vi "GFITS_Dhs_CmdHandling.vi"(0 "imname":string, 1 "fref":u64, 3 "filemsg":string, 5 "command":string, 7 "logfile":path, 9 "data":string, 11 "error in (no error)":errorcluster, 12 "expID":string, 13 "mext":bool, 14 "before expID":string) -> (2 "setref":bool, 4 "nodeID":string, 6 "response":string, 8 "fref out":u64, 10 "impath":string, 15 "error out":errorcluster)   [LabVIEW 2016]
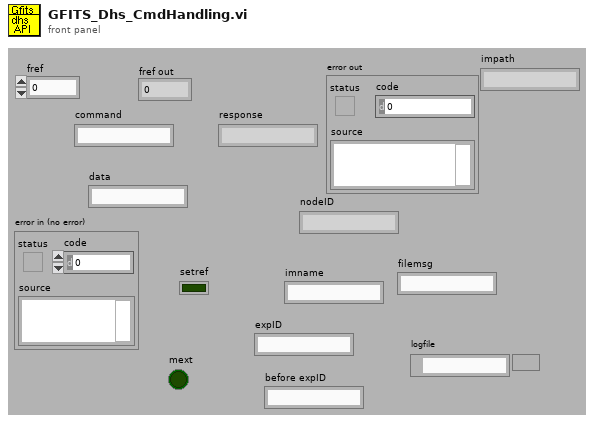
[diagram p1: front panel]
types:
  T1 = typedef "DatabaseHand_RefNum.ctl" = refnum<vi>
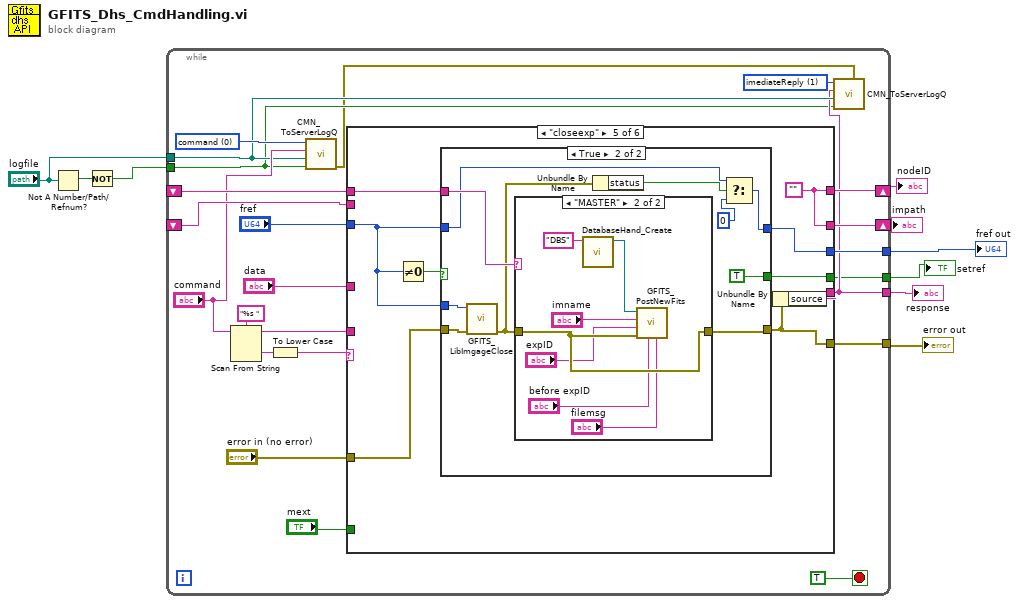
[diagram p0: block diagram]
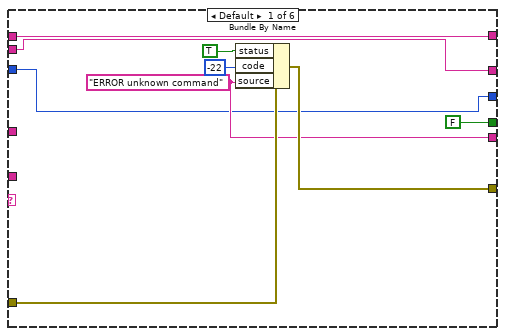
[diagram p2: hidden frame]
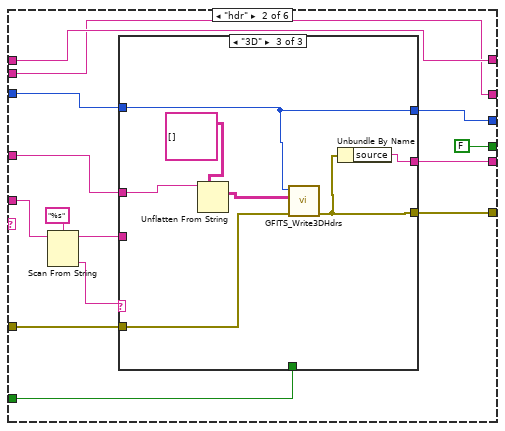
[diagram p3: hidden frame]
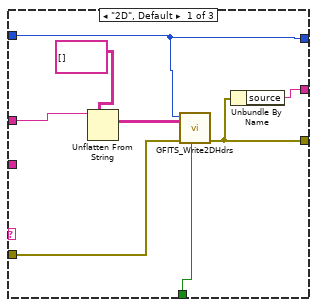
[diagram p4: hidden frame]
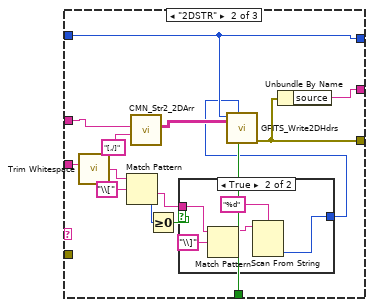
[diagram p5: hidden frame]
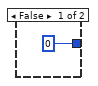
[diagram p6: hidden frame]
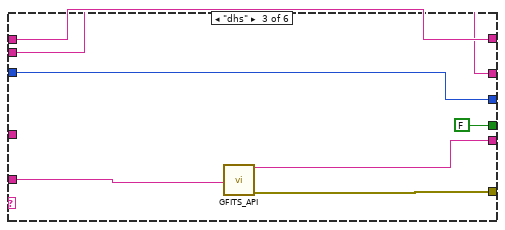
[diagram p7: hidden frame]
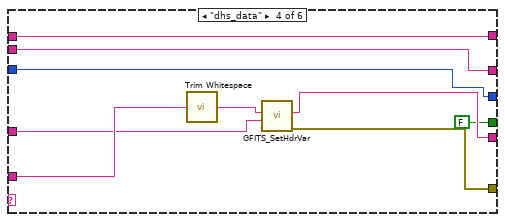
[diagram p8: hidden frame]
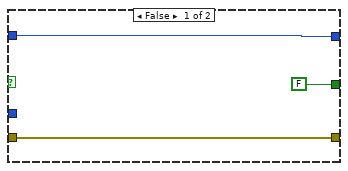
[diagram p9: hidden frame]
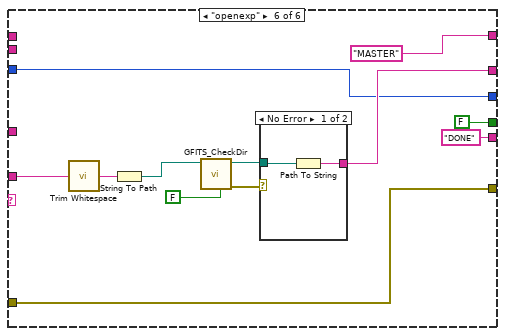
[diagram p11: hidden frame]
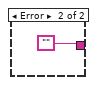
[diagram p12: hidden frame]
diagram:
  n1 = Not A Number/Path/Refnum?(number/path/refnum="logfile") -> (NaN/Path/Refnum?=w4:bool)
  n2 = Not(x=w4) -> (.not. x?=w2:bool)
  n3 = while {
    tunnel: [w26] -> w9
    tunnel: [w13] -> w8
    shift-right: [w23] -> w7
    shift-left: _ -> [w22]
    shift-right: [w21] -> w6
    shift-left: _ -> [w20]
    tunnel: [w19] -> w5
    tunnel: "logfile" -> [w15]
    tunnel: w2 -> [w12]
    tunnel: [w10] -> w1
    stop <- TRUE stop-if-true
    w14 = u16 1 items=["command", "imediateReply", "Callback Reply", "Information", "none"] ("type")
    w17 = u16 0 items=["command", "imediateReply", "Callback Reply", "Information", "none"] ("type")
    n4 = Scan From String(format string="%s ", input string="command") -> (remaining string=w29:string, output 1=w32:string)  [unwired: 2 in, 3 out]
    n5 = To Lower Case(string=w32) -> (all lower case string=w30:string)
    n6 = call "CMN_ToServerLogQ.vi"("Log"=w12, "file"=w15, "string"="command", "type"=w17) -> ("error out"=w11:errorcluster)  [unwired: 2 in, 4 out]
    n7 = case shown="\"closeexp\"" w30 {
      tunnel: w29 -> [_ w53 w96 w105 _ w145]
      tunnel: "data" -> [_ w52 _ w100 _ _]
      tunnel: [w40 w51 w97 w104 w114 w147] -> w26
      tunnel: "error in (no error)" -> [w41 w50 _ _ w115 w147]
      tunnel: [w37 w49 w95 w101 w113 "DONE" ("source")] -> w13
      tunnel: "fref" -> [w34 w48 w92 w99 w109 w138]
      tunnel: [w36 w47 w94 w103 w111 "MASTER"] -> w23
      tunnel: w22 -> [w36 w47 w94 w103 w110 _]
      tunnel: [w35 w46 w93 w102 w111 w139] -> w21
      tunnel: w20 -> [w35 w46 w93 w102 _ _]
      tunnel: [w34 w45 w92 w99 w108 w138] -> w19
      tunnel: "mext" -> [_ w44 _ _ _ _]
      tunnel: [FALSE ("setref") FALSE ("setref") FALSE ("setref") FALSE ("setref") w107 FALSE ("setref")] -> w10
      frame Default {
        w37 = "ERROR unknown command" ("source")
        n8 = Bundle By Name(cluster=w41, "status"=TRUE, "code"=-22, "source"=w37) -> (w40:errorcluster)
      }
      frame "hdr" {
        n9 = Scan From String(format string="%s", input string=w53) -> (remaining string=w43:string, output 1=w54:string)  [unwired: 2 in, 3 out]
        n10 = case shown="\"3D\"" w54 {
          tunnel: w52 -> [w63 w77 w90]
          tunnel: [w59 w74 w86] -> w51
          tunnel: w48 -> [w57 w72 w84]
          tunnel: w50 -> [w60 _ w87]
          tunnel: [w58 w73 w85] -> w49
          tunnel: [w57 w72 w84] -> w45
          tunnel: w44 -> [w56 w71 _]
          tunnel: w43 -> [_ w70 _]
          frame "2D", Default {
            n11 = Unflatten From String(type=string[][] [], binary string=w63) -> (value=w61:string[][])  [unwired: 1 in, 4 out]
            n12 = call "GFITS_Write2DHdrs.vi"("mext"=w56, "error in (no error)"=w60, "keys"=w61, "fref"=w57) -> ("error out"=w59:errorcluster)  [unwired: 1 in, 6 out]
            n13 = Unbundle By Name(w59) -> ("source"=w58:string)
          }
          frame "2DSTR" {
            n14 = call <vilib>:"Trim Whitespace.vi"("string"=w70) -> ("trimmed string"=w69:string)  [unwired: 1 in]
            n15 = Match Pattern(string=w69, regular expression="\\[") -> (after substring=w65:string, offset past match=w67:i32)  [unwired: 3 out]
            n16 = call "CMN_Str2_2DArr.vi"("col separator"="[,/]", "multi line string in"=w77) -> ("array out"=w75:string[][])  [unwired: 9 out]
            n17 = Greater Or Equal To 0?(x=w67) -> (x >= 0?=w66:bool)
            n18 = case shown="True" w66 {
              tunnel: w65 -> [_ w83]
              tunnel: [0 w79] -> w64
              frame False {
              }
              frame True {
                n19 = Match Pattern(string=w83, regular expression="\\]") -> (before substring=w81:string)  [unwired: 4 out]
                n20 = Scan From String(format string="%d", input string=w81) -> (output 1=w79:i32)  [unwired: 2 in, 4 out]
              }
            }
            n21 = call "GFITS_Write2DHdrs.vi"("mext"=w71, "extension"=w64, "keys"=w75, "fref"=w72) -> ("error out"=w74:errorcluster)  [unwired: 1 in, 6 out]
            n22 = Unbundle By Name(w74) -> ("source"=w73:string)
          }
          frame "3D" {
            n23 = Unflatten From String(type=string[][][] [], binary string=w90) -> (value=w88:string[][][])  [unwired: 1 in, 4 out]
            n24 = call "GFITS_Write3DHdrs.vi"("error in (no error)"=w87, "keys"=w88, "fref"=w84) -> ("error out"=w86:errorcluster)  [unwired: 8 out]
            n25 = Unbundle By Name(w86) -> ("source"=w85:string)
          }
        }
      }
      frame "dhs" {
        n26 = call "GFITS_API.vi"("Cmd"=w96) -> ("ImmedReplyString"=w95:string, "error out"=w97:errorcluster)  [unwired: 2 in, 11 out]
      }
      frame "dhs_data" {
        n27 = call <vilib>:"Trim Whitespace.vi"("string"=w105) -> ("trimmed string"=w106:string)  [unwired: 1 in]
        n28 = call "GFITS_SetHdrVar.vi"("data"=w100, "args"=w106) -> ("error out"=w104:errorcluster, "response"=w101:string)  [unwired: 1 in, 7 out]
      }
      frame "closeexp" {
        w111 = ""
        n29 = Not Equal To 0?(x=w109) -> (x != 0?=w112:bool)
        n30 = case shown="True" w112 {
          tunnel: w109 -> [_ w128]
          tunnel: w115 -> [w118 w127]
          tunnel: [w118 w125] -> w114
          tunnel: w110 -> [_ w126]
          tunnel: [w117 w121] -> w108
          tunnel: w109 -> [w117 w120]
          tunnel: [FALSE ("setref") TRUE ("setref")] -> w107
          frame False {
          }
          frame True {
            n31 = call "GFITS_LibImgageClose.vi"("error in (no error)"=w127, "fd"=w128) -> ("error out"=w124:errorcluster)  [unwired: 1 in, 8 out]
            n32 = case shown="\"MASTER\"" w126 {
              tunnel: w124 -> [w129 w136]
              tunnel: [w129 w136] -> w125
              frame Default {
              }
              frame "MASTER" {
                n33 = call "DatabaseHand_Create.vi"("Name"="DBS") -> ("Database RefNum out"=w134:T1)  [unwired: 1 in, 9 out]
                n34 = call "GFITS_PostNewFits.vi"("filemsg"="filemsg", "before_expID"="before expID", "error in"=w136, "expID"="expID", "image name"="imname", "Database RefNum in"=w134) -> ()  [unwired: 6 out]
              }
            }
            n35 = Unbundle By Name(w124) -> ("status"=w123:bool)
            n36 = Select(t=w120, s=w123, f=u64 0 ("fref out")) -> (s? t:f=w121:u64)
          }
        }
        n37 = Unbundle By Name(w114) -> ("source"=w113:string)
      }
      frame "openexp" {
        n38 = call <vilib>:"Trim Whitespace.vi"("string"=w145) -> ("trimmed string"=w143:string)  [unwired: 1 in]
        n39 = String To Path(string=w143) -> (path=w144:path)
        n40 = call "GFITS_CheckDir.vi"("create?"=FALSE ("Generate Error?"), "impath in"=w144) -> ("error out"=w141:errorcluster, "impath out"=w140:path)  [unwired: 1 in, 7 out]
        n41 = case shown="No Error" w141 {
          tunnel: w140 -> [w150 _]
          tunnel: [w149 ""] -> w139
          frame No Error {
            n42 = Path To String(path=w150) -> (string=w149:string)
          }
          frame Error {
          }
        }
      }
    }
    n43 = call "CMN_ToServerLogQ.vi"("error in (no error)"=w11, "Log"=w12, "file"=w15, "string"=w13, "type"=w14) -> ()  [unwired: 1 in, 5 out]
  }
  "response" <- w8
  "error out" <- w9
  "nodeID" <- w7
  "impath" <- w6
  "fref out" <- w5
  "setref" <- w1
